vi "ControlDeviation (SubVI).vi"(0 "Set Value":dbl format="%#_13g", 1 "Actual Value":dbl format="%#_13g", 4 "Tolerance [%]":dbl format="%#_13g") -> (7 "Deviation [%]":dbl, 8 "In Tolerance?":bool)   [LabVIEW 2015]
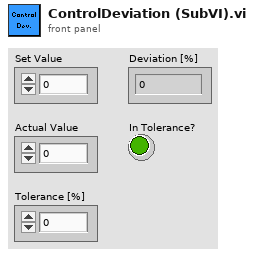
[diagram p1: front panel]
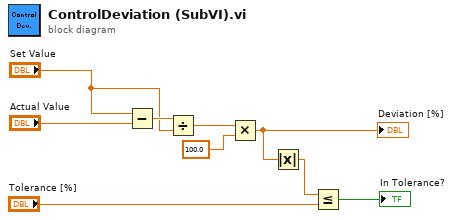
[diagram p0: block diagram]
diagram:
  n1 = Subtract(x="Set Value", y="Actual Value") -> (x-y=w5:dbl)
  n2 = Divide(x=w5, y="Set Value") -> (x/y=w3:dbl)
  n3 = Multiply(x=w3, y=100.0) -> (x*y=w8:dbl)
  "Deviation [%]" <- w8
  n4 = Absolute Value(x=w8) -> (abs(x)=w9:dbl)
  n5 = Less Or Equal?(x=w9, y="Tolerance [%]") -> (x <= y?=→"In Tolerance?":bool)
